vi "User Authentication Schemes.vi"(8 "Error In":errorcluster, 10 "Username":string, 11 "Session In":refnum<class "Session.lvclass">) -> (0 "Error Out":errorcluster, 2 "Supported Schemes":T1[](array[typedef]), 3 "Sesssion Out":refnum<class "Session.lvclass">)   [LabVIEW 2017, in "Toolkit.lvlib" / "Session.lvclass"]
uses:
  Session.lvclass
  Typedefs/User Authentication Schemes.ctl
  Session.lvclass/Session.ctl
  Toolkit.lvlib
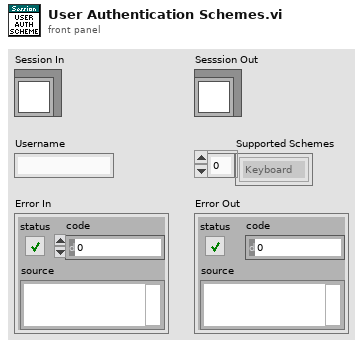
[diagram p1: front panel]
types:
  T1 = typedef "Toolkit.lvlib/Session.lvclass/User Authentication Schemes.ctl" = enum16{"Keyboard", "Password", "Public Key"}
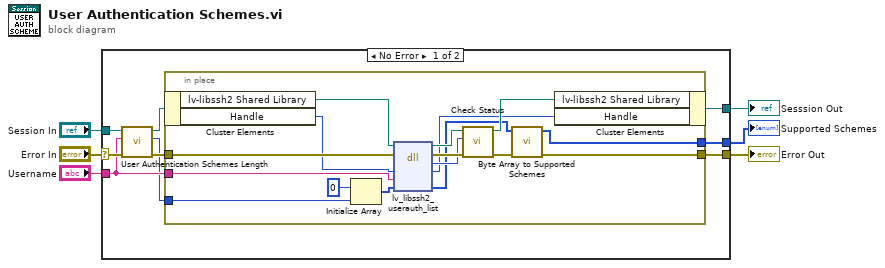
[diagram p0: block diagram]
diagram:
  n1 = case shown="No Error" "Error In" {
    selector: "Error In" -> [w13 w33]
    tunnel: [w14 w33] -> w5
    tunnel: "Session In" -> [w11 w32]
    tunnel: [w15 w32] -> w3
    tunnel: "Username" -> [w9 _]
    tunnel: [w7 _] -> w1
    frame No Error {
      n2 = call "User Authentication Schemes Length.vi"("Error In"=w13, "Username"=w9, "Session In"=w11) -> ("Error Out"=w12:errorcluster, "Length"=w8:i32, "Sesssion Out"=w10:refnum<class "Session.lvclass">)  [unwired: 6 in]
      n3 = in-place {
        in-place-border: w12 -> [w27]
        in-place-border: [w16] -> w14
        in-place-border: w9 -> [w25]
        in-place-border: w8 -> [w22]
        in-place-border: [w18] -> w7
        n4 = in-place-cluster #1(w10) -> ("lv-libssh2 Shared Library"=w31:path, "Handle"=w24:u64)
        n5 = Initialize Array(u8 0, w22) -> (w20:u8[])
        n6 = dll-call lib="D:/Users/cfield/Code/Field R&D Services/SSH/LV-LIBSSH2/LabVIEW/trunk/src/Toolkit/Support/lv-libssh2.dll" fn="lv_libssh2_userauth_list"(path in=w31, error in=w27, "session"=w24, "username"=w25, "buffer"=w20) -> (path out=w29:path, error out=w30:errorcluster, "result"=w28:i32, "session"=w23:u64, "buffer"=w19:u8[])  [unwired: 2 in]
        n7 = call "Check Status.vi"("Error In"=w30, "Status"=w28, "lv-libssh2 Shared Library In"=w29) -> ("Error Out"=w17:errorcluster, "lv-libssh2 Shared Library Out"=w26:path)  [unwired: 7 in]
        n8 = call "Byte Array to Supported Schemes.vi"("Error In"=w17, "Buffer"=w19) -> ("Error Out"=w16:errorcluster, "Supported Schemes"=w18:T1[])  [unwired: 8 in]
        n9 = in-place-cluster #1("lv-libssh2 Shared Library"=w26, "Handle"=w23) -> (w15:refnum<class "Session.lvclass">)
      }
    }
    frame Error {
    }
  }
  "Sesssion Out" <- w3
  "Error Out" <- w5
  "Supported Schemes" <- w1
